vi "Fault Code Lookup.vi"(11 "Fault Code":u64) -> (3 "Active Faults":string[](array[string]))   [LabVIEW 2023]
uses:
  Types/ERROR_GLOBAL.ctl
panel:
  in  "ERROR_GLOBAL":T1 items=["ERROR_GLOB_EMO_GLOBAL"=0, "ERROR_GLOB_EMO_BUTTON_PRESSED"=1, "ERROR_GLOB_USER"=2, "ERROR_GLOB_PM"=3, "ERROR_GLOB_GRID"=4, "ERROR_GLOB_VOLTAGE_DCBUS_OUT_OF_BOUNDS"=6, "ERROR_GLOB_VOLTAGE_OUTPUT_HIGH"=7, "ERROR_GLOB_VOLTAGE_OUTPUT_LOW"=8, "ERROR_GLOB_VOLTAGE_OUTPUT_UNBALANCE"=9, "ERROR_GLOB_CURRENT_OUTPUT_HIGH"=10, "ERROR_GLOB_SYS_OVERTEMPERATURE"=13, "ERROR_GLOB_SYS_HW"=14, "ERROR_GLOB_SYS_COMM"=15, "ERROR_GLOB_SYNC_AND_CONNECT"=16, "ERROR_GLOB_SP"=20, "ERROR_GLOB_SP_TRACKING"=21, "ERROR_GLOB_CONFIG"=23, "ERROR_GLOB_REG_SYS"=27, "ERROR_GLOB_REG_GRID"=28, "ERROR_GLOB_REG_AFE1"=29, "ERROR_GLOB_REG_AFE2"=30, "ERROR_GLOB_REG_DC"=31]
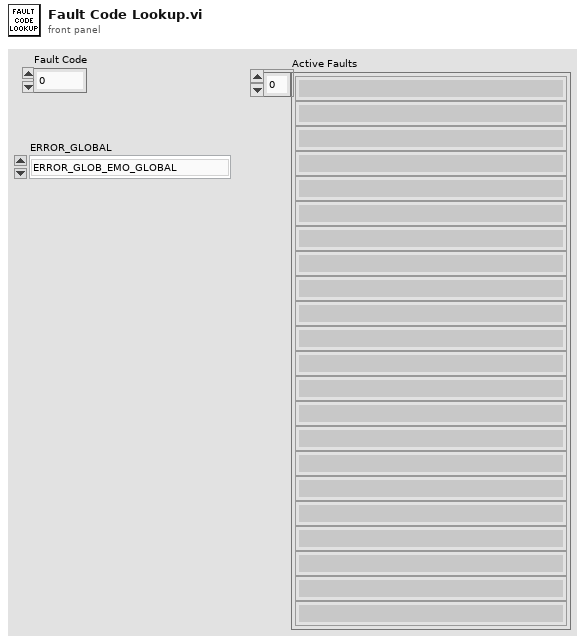
[diagram p1: front panel]
types:
  T1 = typedef "ERROR_GLOBAL.ctl" = u32
  T2 = typedef "LVStringsAndValuesArrayTypeDef_U32.ctl" = cluster{"String":string, "Value":u32}[]
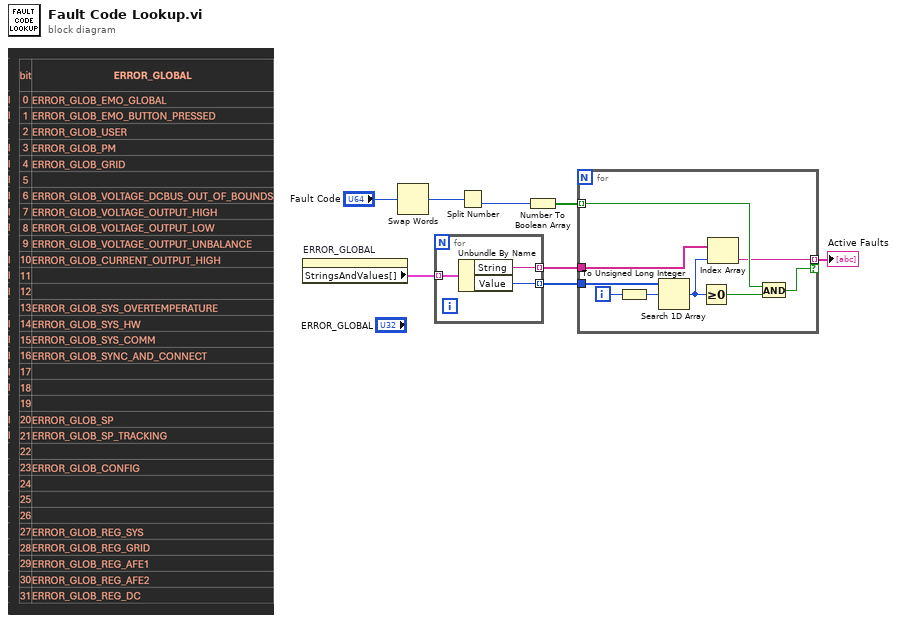
[diagram p0: block diagram]
diagram:
  n1 = property on="ERROR_GLOBAL" class="Ring (strict)"() -> ("StringsAndValues[]"=w8:T2)  [unwired: 2 in, 2 out]
  n2 = Swap Words(1:"Fault Code") -> (0:w2:u64)
  n3 = for {
    tunnel: w8 -> [w11] mode=indexing
    tunnel: [w10] -> w6 mode=indexing
    tunnel: [w9] -> w7 mode=indexing
    n4 = Unbundle By Name(w11) -> ("String"=w10:string, "Value"=w9:u32)
  }
  n5 = Split Number(x=w2) -> (lo(x)=w1:u32)  [unwired: 1 out]
  n6 = Number To Boolean Array(number=w1) -> (Boolean array=w4:bool[])
  n7 = for {
    tunnel: w4 -> [w14] mode=indexing
    tunnel: w7 -> [w20]
    tunnel: w6 -> [w15]
    tunnel: [w13] -> w5 mode=indexing if=w12
    i -> [w19]
    n8 = To Unsigned Long Integer(number=w19) -> (unsigned 32bit integer=w18:u32)
    n9 = Search 1D Array(1D array=w20, element=w18) -> (index of element=w16:i32)  [unwired: 1 in]
    n10 = Greater Or Equal To 0?(x=w16) -> (x >= 0?=w17:bool)
    n11 = Index Array(array=w15, index=w16) -> (element=w13:string)
    n12 = And(x=w14, y=w17) -> (x .and. y?=w12:bool)
  }
  "Active Faults" <- w5
